vi "enum.vi"() -> ()   [LabVIEW 2019]
panel:
  in  "Enum":enum16{"FUCKING SLAVE", "FULL MASTER", "BILLY"}(ring)
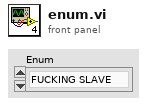
[diagram p1: front panel]
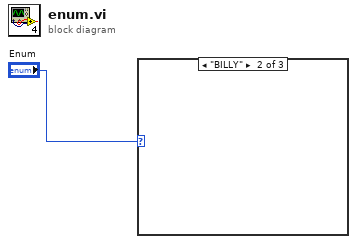
[diagram p0: block diagram]
diagram:
  n1 = case shown="\"BILLY\"" "Enum" {
    frame "FUCKING SLAVE", Default {
    }
    frame "BILLY" {
    }
    frame "FULL MASTER" {
    }
  }
